vi "configure.vi"(8 "error in (no error)":errorcluster, 11 "GenericPlugin in":refnum<class "DataCollectionMG091001IntrinsicImaging.lvclass">) -> (0 "error out":errorcluster, 3 "GenericPlugin out":refnum<class "DataCollectionMG091001IntrinsicImaging.lvclass">)   [LabVIEW 2010, in "DataCollectionMG091001IntrinsicImaging.lvclass"]
doc: "The dynamic dispatch version of this VI loads and displays the configuration file associated with the plug-in object. The user modify and save the configuration data."
uses:
  DataCollectionMG091001IntrinsicImaging.lvclass
  DataCollectionMG091001IntrinsicImaging.lvclass/DataCollectionMG091001IntrinsicImaging.ctl
  common/classes/ErrorController/ErrorController/class_data.vi
  common/classes/GenericComponent/GenericComponent/GenericComponent.lvclass
  common/classes/ErrorController/ErrorController/ErrorController.lvclass
panel:
  in  "Tab Control":T1(tab)
  in  "image multiplication factor":dbl
  out "configuration":string
  in  "cancel button":bool
  in  "save button":bool
  # "Configure DataCollectionMG091001IntrinsicImaging"
  # "The task of the DataCollectionMG091001IntrinsicImaging component is to receive individiual images, to calculate difference images, to calculate average images and to store these images to disk."
  # "Intrinsic signals are typical very small fractional values (in the order of 0.001). Since images are saved in a UInt16 format, up-scaling by a certain multiplication factor is required.\n\nExample: In order to losslessly store values with a maximal size of 0.006 in a UInt16 TIFF file (which has a range of 0-65535), they have to be multiplied by 1E7.\n\nImportant: In order to prevent a range overflow for large signal values, the factor should not be chosen too high. I.e., in the example above, a value of 1E6 would be saver."
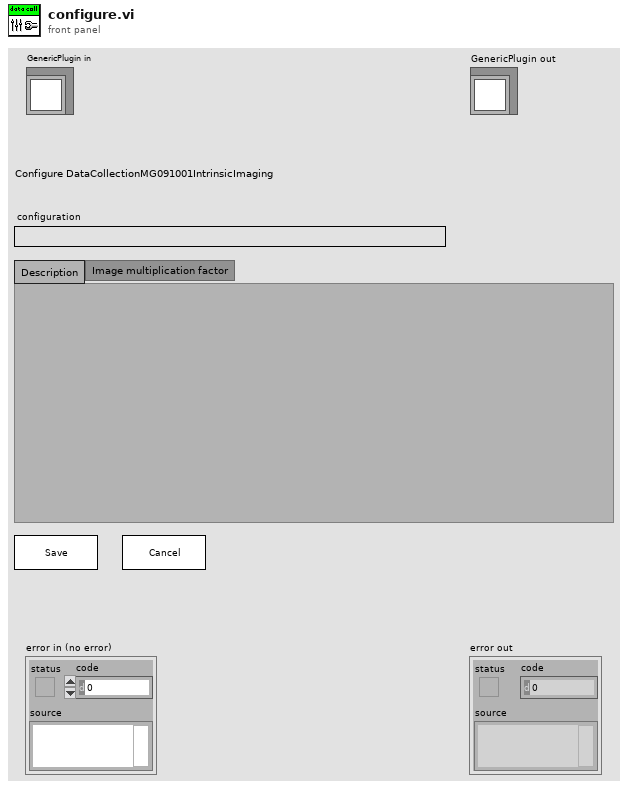
[diagram p1: front panel]
types:
  T1 = enum32{"Description", "Image multiplication factor"}
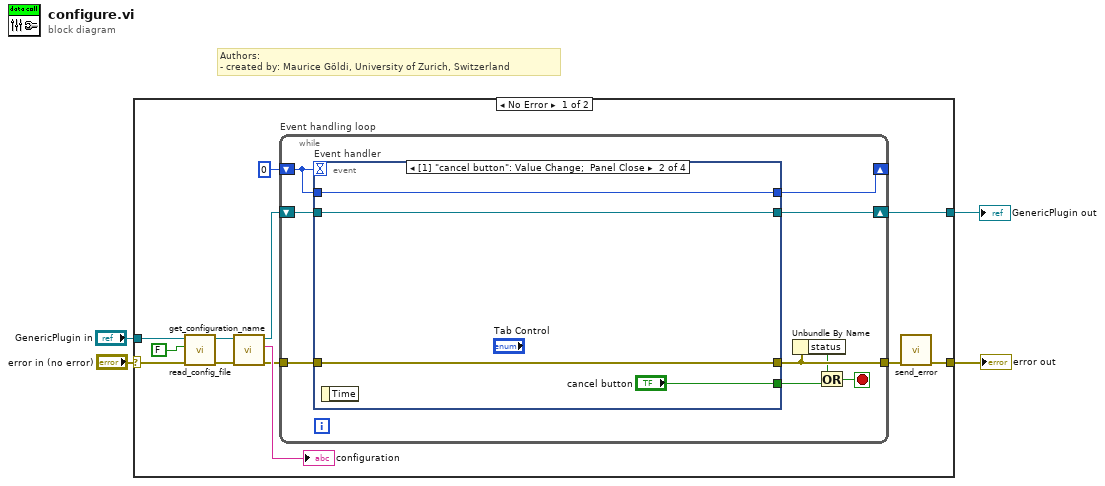
[diagram p0: block diagram]
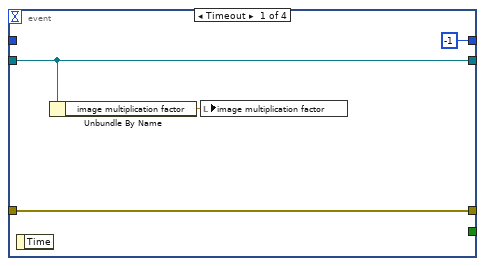
[diagram p2: hidden frame]
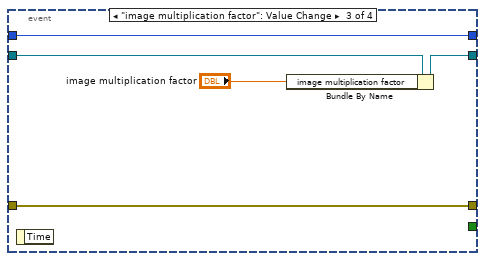
[diagram p3: hidden frame]
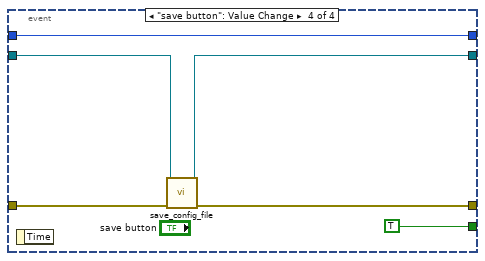
[diagram p4: hidden frame]
diagram:
  # "Authors: \n- created by: Maurice Göldi, University of Zurich, Switzerland"
  n1 = case shown="No Error" "error in (no error)" {
    selector: "error in (no error)" -> [w16 w46]
    tunnel: [w6 w46] -> w3
    tunnel: "GenericPlugin in" -> [w14 w45]
    tunnel: [w7 w45] -> w1
    frame No Error {
      n2 = call-dynamic "read_config_file.vi"("error in (no error)"=w16, "force load?"=FALSE, "GenericPlugin in"=w14) -> ("error out"=w13:errorcluster, "GenericPlugin out"=w12:refnum<class "DataCollectionMG091001IntrinsicImaging.lvclass">)  [unwired: 7 in]
      n3 = call "get_configuration_name.vi"("error in (no error)"=w13, "GenericPlugin.lvclass in"=w12) -> ("error out"=w9:errorcluster, "configuration name"=→"configuration":string, "GenericPlugin.lvclass out"=w8:refnum<class "DataCollectionMG091001IntrinsicImaging.lvclass">)  [unwired: 7 in]
      n4 = while "Event handling loop" {
        shift-right: [w25] -> _
        shift-left: 0 -> [w21]
        shift-right: [w23] -> w7
        shift-left: w8 -> [w22]
        tunnel: w9 -> [w24]
        tunnel: [w20] -> w5
        stop <- w18 stop-if-true
        n5 = event "Event handler" shown="[1] \"cancel button\": Value Change;  Panel Close" {
          selector: _ -> [_ _ _ _]
          dyn-events: _ -> [_ _ _ _]
          timeout: w21 -> [_ _ _ _]
          tunnel: w21 -> [_ w33 w38 w44]
          tunnel: [-1 w33 w38 w44] -> w25
          tunnel: w24 -> [w28 w32 w37 w42]
          tunnel: [w28 w32 w37 w41] -> w20
          tunnel: [w27 w30 w35 w39] -> w23
          tunnel: w22 -> [w27 w30 w36 w40]
          tunnel: [_ "cancel button" _ TRUE] -> w17
          event Timeout {
            n6 = event-data() -> ()  [unwired: 1 in, 1 out]
            n7 = Unbundle By Name(w27) -> ("image multiplication factor"=w26:dbl)
            n8 = local write "image multiplication factor"(w26) -> ()
          }
          event "cancel button": Value Change; Panel Close {
            n9 = event-data() -> ()  [unwired: 1 in, 1 out]
          }
          event "image multiplication factor": Value Change {
            n10 = event-data() -> ()  [unwired: 1 in, 1 out]
            n11 = Bundle By Name(cluster=w36, "image multiplication factor"="image multiplication factor") -> (w35:refnum<class "DataCollectionMG091001IntrinsicImaging.lvclass">)
          }
          event "save button": Value Change {
            n12 = event-data() -> ()  [unwired: 1 in, 1 out]
            n13 = call-dynamic "save_config_file.vi"("error in (no error)"=w42, "GenericPlugin in"=w40) -> ("error out"=w41:errorcluster, "GenericPlugin out"=w39:refnum<class "DataCollectionMG091001IntrinsicImaging.lvclass">)  [unwired: 8 in]
          }
        }
        n14 = Unbundle By Name(w20) -> ("status"=w19:bool)
        n15 = Or(x=w19, y=w17) -> (x .or. y?=w18:bool)
      }
      n16 = call "send_error.vi"("error in (no error)"=w5) -> ("error out"=w6:errorcluster)  [unwired: 10 in]
    }
    frame Error {
    }
  }
  "error out" <- w3
  "GenericPlugin out" <- w1
